vi "Sort Channel Array.vi"(10 "Sort":T1, 11 "channels":refnum<class "TBM channel.lvclass">[](array[class])) -> (3 "Array":refnum<class "TBM channel.lvclass">[](array[class]))   [LabVIEW 2015, in "GraphViz Mapping Visualizer.lvlib"]
doc: "Sorrts channels by name (if enabled) in ascending or descending order."
uses:
  GraphViz Mapping Visualizer.lvlib
  <vilib>/NI/Tag Bus Module Framework/channel/TBM channel.lvclass
  Sort Options.ctl
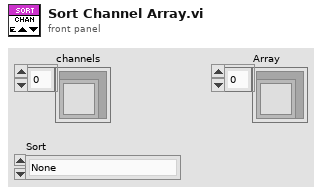
[diagram p1: front panel]
types:
  T1 = typedef "GraphViz Mapping Visualizer.lvlib/Sort Options.ctl" = enum16{"None", "All Ascending", "All Descending", "Channel Type Ascending", "Channel Type Descending"}
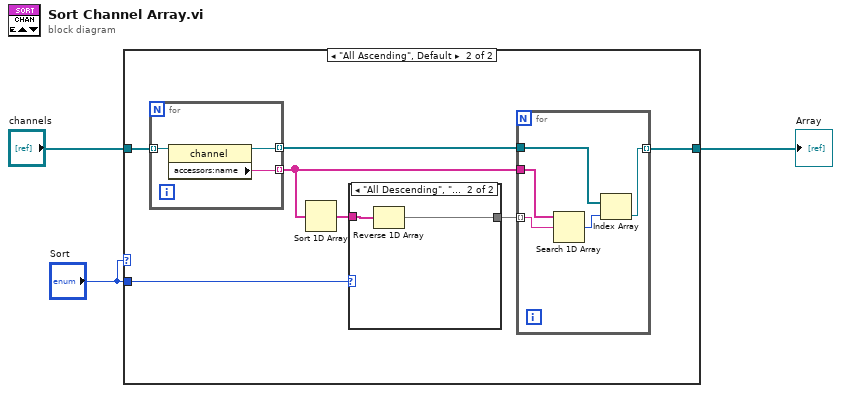
[diagram p0: block diagram]
diagram:
  n1 = case shown="\"All Ascending\", Default" "Sort" {
    tunnel: [w4 w11] -> w3
    tunnel: "Sort" -> [_ w6]
    tunnel: "channels" -> [w4 w5]
    frame "None" {
    }
    frame "All Ascending", Default {
      n2 = for {
        tunnel: w5 -> [w22] mode=indexing
        tunnel: [w21] -> w10 mode=indexing
        tunnel: [w20] -> w8 mode=indexing
        n3 = property class="channel"(reference=w22) -> (reference out=w20:refnum<class "TBM channel.lvclass">, "accessors:name"=w21:string)  [unwired: 1 in, 1 out]
      }
      n4 = Sort 1D Array(array=w10) -> (sorted array=w7:string[])
      n5 = case shown="\"All Descending\", \"Channel Type Descending\"" w6 {
        tunnel: w7 -> [w17 w19]
        tunnel: [w17 w18] -> w9
        frame Default {
        }
        frame "All Descending", "Channel Type Descending" {
          n6 = Reverse 1D Array(array=w19) -> (reversed array=w18:string[])
        }
      }
      n7 = for {
        tunnel: w8 -> [w15]
        tunnel: w9 -> [w12] mode=indexing
        tunnel: w10 -> [w13]
        tunnel: [w14] -> w11 mode=indexing
        n8 = Search 1D Array(1D array=w13, element=w12) -> (index of element=w16:i32)  [unwired: 1 in]
        n9 = Index Array(array=w15, index=w16) -> (element=w14:refnum<class "TBM channel.lvclass">)
      }
    }
  }
  "Array" <- w3
